vi "CS4_read.vi"(3 "error in":errorcluster, 5 "address string":string) -> (0 "error out":errorcluster, 1 "Sweep Set point (Low)":string, 2 "Sweep Set point (high)":string, 4 "Real Field":string)   [LabVIEW 2012]
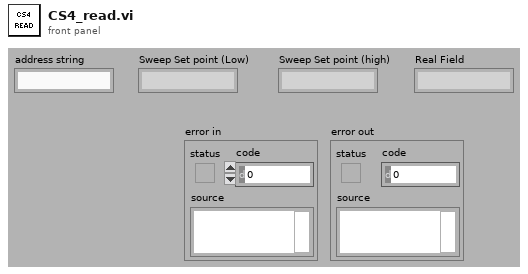
[diagram p1: front panel]
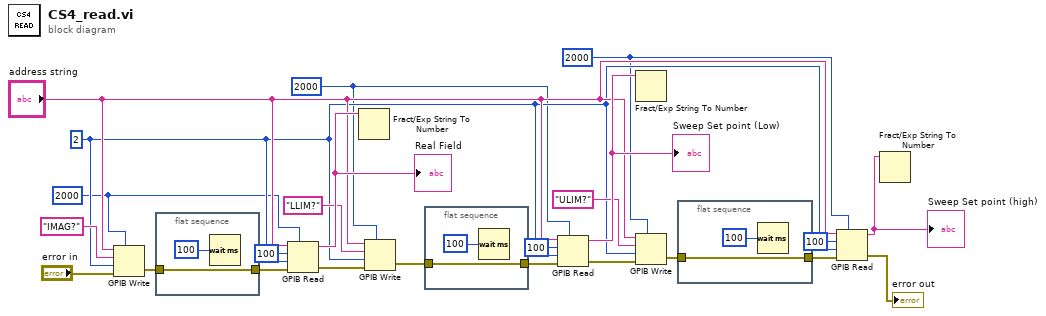
[diagram p0: block diagram]
diagram:
  w5 = 2000 ("timeout ms (488.2 global)")
  w6 = 2000 ("timeout ms (488.2 global)")
  w7 = 2000 ("timeout ms (488.2 global)")
  w8 = i16 2 ("mode (0)")
  n1 = GPIB Write(0:"address string", 1:"IMAG?" ("data"), 2:w8, 3:"error in", 4:w5) -> (6:w23:errorcluster)  [unwired: 1 out]
  n2 = flat-sequence {
    tunnel: w23 -> [w25]
    tunnel: [w25] -> w22
    frame #0 {
      n3 = Wait (ms)(milliseconds to wait=u32 100) -> ()  [unwired: 1 out]
    }
  }
  n4 = GPIB Read(0:"address string", 1:100 ("byte count"), 2:w8, 3:w22, 4:w5) -> (5:w21:string, 7:w15:errorcluster)  [unwired: 1 out]
  "Real Field" <- w21
  n5 = Fract/Exp String To Number(string=w21) -> ()  [unwired: 3 in, 2 out]
  n6 = GPIB Write(0:"address string", 1:"LLIM?" ("data"), 2:w8, 3:w15, 4:w6) -> (6:w19:errorcluster)  [unwired: 1 out]
  n7 = flat-sequence {
    tunnel: w19 -> [w27]
    tunnel: [w27] -> w18
    frame #0 {
      n8 = Wait (ms)(milliseconds to wait=u32 100) -> ()  [unwired: 1 out]
    }
  }
  n9 = GPIB Read(0:"address string", 1:100 ("byte count"), 2:w8, 3:w18, 4:w6) -> (5:w17:string, 7:w10:errorcluster)  [unwired: 1 out]
  "Sweep Set point (Low)" <- w17
  n10 = Fract/Exp String To Number(string=w17) -> ()  [unwired: 3 in, 2 out]
  n11 = GPIB Write(0:"address string", 1:"ULIM?" ("data"), 2:w8, 3:w10, 4:w7) -> (6:w13:errorcluster)  [unwired: 1 out]
  n12 = flat-sequence {
    tunnel: w13 -> [w29]
    tunnel: [w29] -> w12
    frame #0 {
      n13 = Wait (ms)(milliseconds to wait=u32 100) -> ()  [unwired: 1 out]
    }
  }
  n14 = GPIB Read(0:"address string", 1:100 ("byte count"), 2:w8, 3:w12, 4:w7) -> (5:w11:string, 7:→"error out":errorcluster)  [unwired: 1 out]
  "Sweep Set point (high)" <- w11
  n15 = Fract/Exp String To Number(string=w11) -> ()  [unwired: 3 in, 2 out]
